vi "Clear Hardware.vi"(2 "error in (no error)":errorcluster, 3 "Master Device in":refnum<class "Master Device.lvclass"> caption="Device in") -> (0 "error out":errorcluster, 1 "Master Device out":refnum<class "Master Device.lvclass"> caption="Device out")   [LabVIEW 2013, in "Master Device.lvclass"]
doc: "This VI resets any necessary hardware so that the device will be ready for the next run."
uses:
  Master Device.lvclass
  Device/Device.lvclass
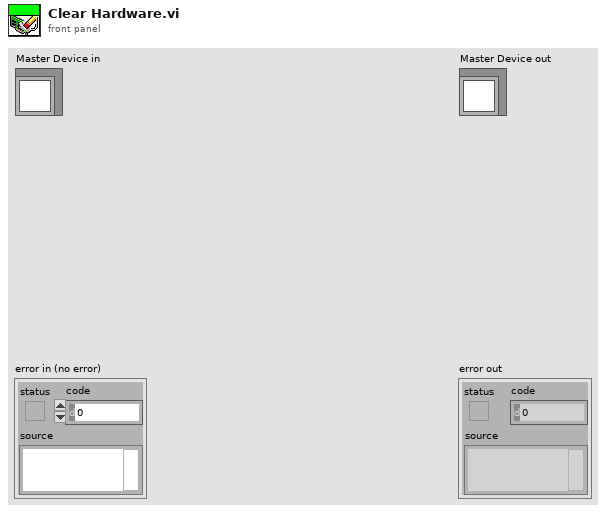
[diagram p1: front panel]
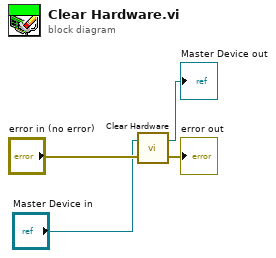
[diagram p0: block diagram]
diagram:
  n1 = call-parent "Clear Hardware.vi"("error in (no error)"="error in (no error)", "Device in"="Master Device in") -> ("error out"=→"error out":errorcluster, "Device out"=→"Master Device out":refnum<class "Master Device.lvclass">)
